vi "read station LIN config.vi"(0 "configuration file path in":path, 1 "lin channel count":i32=1, 5 "station idx":i32, 9 "ldf file name":string="CD701_CEM_LIN3_20230222", 11 "error in":errorcluster, 12 "NAD":u8) -> (3 "XNET LIN":bool, 4 "configuration file path out":path, 8 "LIN INFO":T1={"Toolkit Type"=enum."Inalfa LIN", "NAD"=36, "Inalfa LIN"={"Master Frame(3C)"="MasterReq\nSPA3414_ConfigurationsCMAGeely_CEMCALYPSOSDB34XX0Cfg_LIN3_190709_", "Slave Frame(3D)"="SlaveResp\nSPA3414_ConfigurationsCMAGeely_CEMCALYPSOSDB34XX0Cfg_LIN3_190709_", "Request Schedule"="CEMLIN3DiagRequestSchedule\nSPA3414_ConfigurationsCMAGeely_CEMCALYPSOSDB34XX0Cfg_LIN3_190709_", "Response Schedule"="CEMLIN3DiagResponseSchedule\nSPA3414_ConfigurationsCMAGeely_CEMCALYPSOSDB34XX0Cfg_LIN3_190709_", "Frame Write SCU"="", "Frame Read SCU"="", "LIN Name"=""}, "ADCS LIN"={"Port"="", "HW select"=0, "XNET Cluster"="NIXNET_exampleLDF", "ByteCmd Path"=path "C:/Labview Code/System/ByteCmdConfig.txt"}, "TS LIN"={"ref info"=refnum, "LIN Channel"=0, "ByteCmd Path"=path "C:/Labview Code/System/ByteCmdConfig.txt"}} {"NAD" format="%.0x"; "ADCS LIN"."HW select" items=["NI-XNET", "NI-CAN"]}, 15 "error out":errorcluster)   [LabVIEW 2018]
uses:
  02.Type Def's/station LIN config.ctl
  03.Inalfa LIN/LIN Device.ctl
  <vilib>/CMC.AME/Inalfa ADCS/Ctl'Def/ADCS_LIN info.ctl
  C:/Program Files (x86)/National Instruments/LabVIEW 2018/vi.lib/CMC.AME/Inalfa TS LIN/TOSUN/TSMaster/bin/Interop.TSMasterAPI.dll
  Program Files (x86)/National Instruments/LabVIEW 2018/vi.lib/CMC.AME/Inalfa TS LIN/TOSUN/TSMaster/bin/Interop.TSMasterAPI.dll
  05.UserVI's/file io/ini/type defs/ini file actions.ctl
  05.UserVI's/file io/ini/type defs/ini entry types.ctl
  05.UserVI's/file io/ini/type defs/ini entry.ctl
  05.UserVI's/file io/ini/type defs/ini entry value.ctl
panel:
  out "LIN Device Name":string
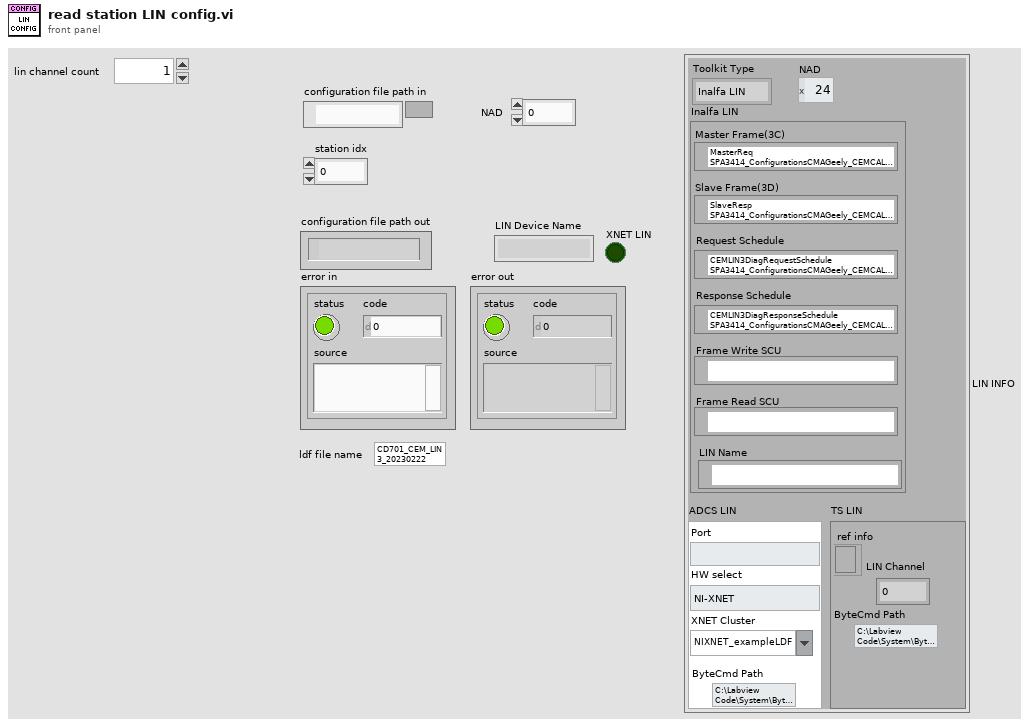
[diagram p1: front panel]
types:
  T1 = typedef "station LIN config.ctl" = cluster{"Toolkit Type":enum16{"Inalfa LIN", "ADCS LIN", "TS LIN"}, "NAD":u8, "Inalfa LIN":T2, "ADCS LIN":T3, "TS LIN":cluster{"ref info":refnum<k24>, "LIN Channel":i32, "ByteCmd Path":path}}
  T2 = typedef "LIN Device.ctl" = cluster{"Master Frame(3C)":refnum<k21>, "Slave Frame(3D)":refnum<k21>, "Request Schedule":refnum<k21>, "Response Schedule":refnum<k21>, "Frame Write SCU":refnum<k21>, "Frame Read SCU":refnum<k21>, "LIN Name":refnum<k21>}
  T3 = typedef "ADCS_LIN info.ctl" = cluster{"Port":string, "HW select":u16, "XNET Cluster":string, "ByteCmd Path":path}
  T4 = typedef "ini file actions.ctl" = enum16{"read ini", "write ini"}
  T5 = typedef "ini entry.ctl" = cluster{"section":string, "key":string, "type":T6, "default value":T7}
  T6 = typedef "ini entry types.ctl" = enum16{"Boolean", "Double", "I32", "Path", "String", "U32"}
  T7 = typedef "ini entry value.ctl" = cluster{"Boolean":bool, "Dbl":dbl, "I32":i32, "Path":path, "String":string, "U32":u32}
  T8 = cluster{"status":bool, "code":i32, "error desp":string}
  T9 = cluster{"Ref out":refnum<k24>, "station idx":i32, "appended path":path}
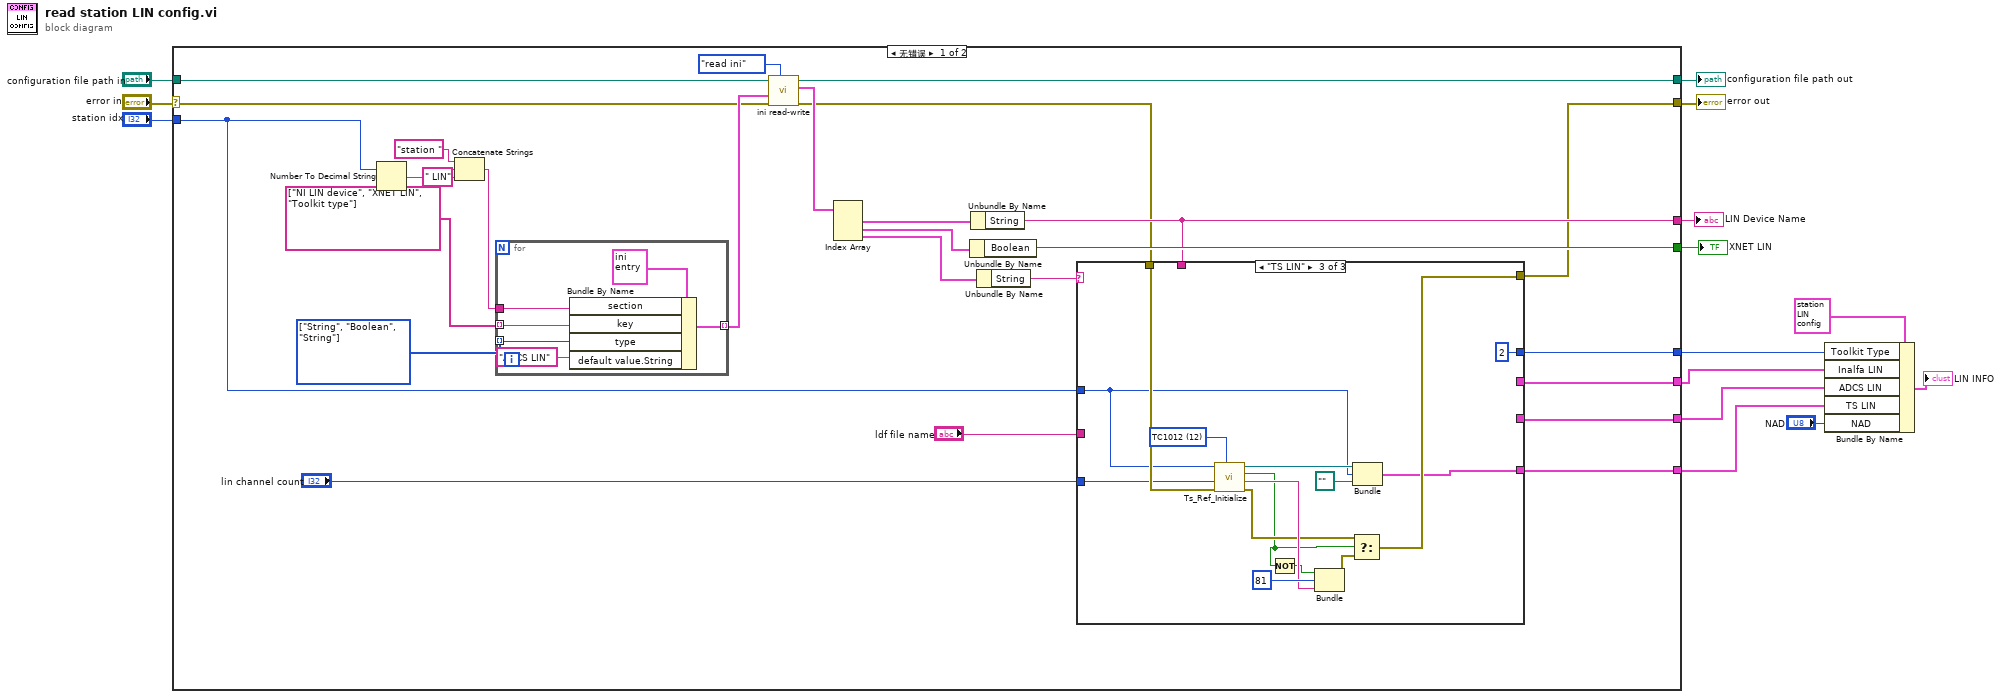
[diagram p0: block diagram]
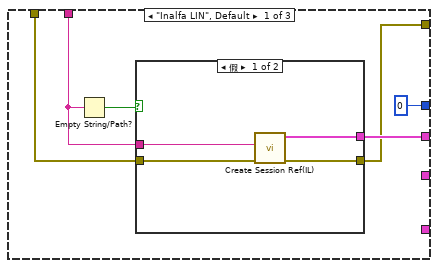
[diagram p2: hidden frame]
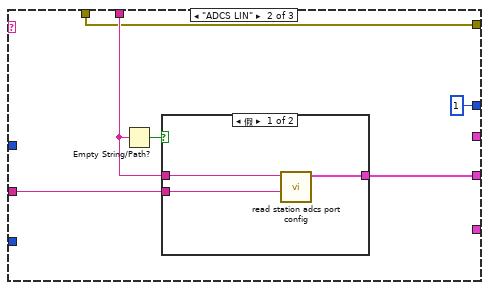
[diagram p4: hidden frame]
diagram:
  n1 = case shown="无错误" "error in" {
    selector: "error in" -> [w32 w84]
    tunnel: "configuration file path in" -> [w41 w83]
    tunnel: [w18 w83] -> w13
    tunnel: [w22 w84] -> w12
    tunnel: "station idx" -> [w16 _]
    tunnel: [w25 _] -> w9
    tunnel: [w28 _] -> w8
    tunnel: [w24 _] -> w6
    tunnel: [w21 _] -> w5
    tunnel: [w19 _] -> w2
    tunnel: [w17 _] -> w3
    frame No Error {
      w34 = T6[] [enum."String", enum."Boolean", enum."String"] items=["Boolean", "Double", "I32", "Path", "String", "U32"]
      n2 = Number To Decimal String(number=w16) -> (decimal integer string=w37:string)  [unwired: 1 in]
      n3 = Concatenate Strings("station ", w37, " LIN" ("string")) -> (w36:string)
      n4 = for {
        tunnel: w36 -> [w81]
        tunnel: string[] ["NI LIN device", "XNET LIN", "Toolkit type"] -> [w80] mode=indexing
        tunnel: w34 -> [w79] mode=indexing
        tunnel: [w78] -> w33 mode=indexing
        n5 = Bundle By Name(cluster=T5 {"section"="", "key"="", "type"=enum."Boolean", "default value"={"Boolean"=FALSE, "Dbl"=0.0, "I32"=0, "Path"=path "", "String"="", "U32"=0}}, "section"=w81, "key"=w80, "type"=w79, "default value.String"="ADCS LIN") -> (w78:T5)
      }
      n6 = call "ini read-write.vi"("action"=ini_file_actions."read ini", "error in (no error)"=w32, "ini entry descriptors"=w33, "configuration file path"=w41) -> ("error out"=w23:errorcluster, "values out"=w39:T7[], "configuration file path out"=w18:path)  [unwired: 5 in]
      n7 = Index Array(array=w39) -> (element #1=w30:T7, element #2=w29:T7, element #3=w27:T7)  [unwired: 3 in]
      n8 = Unbundle By Name(w29) -> ("Boolean"=w28:bool)
      n9 = Unbundle By Name(w30) -> ("String"=w25:string)
      n10 = Unbundle By Name(w27) -> ("String"=w26:string)
      n11 = case shown="\"TS LIN\"" w26 {
        tunnel: w25 -> [w46 w58 _]
        tunnel: [w47 _ _] -> w24
        tunnel: w23 -> [w44 w54 w68]
        tunnel: [w43 w54 w73] -> w22
        tunnel: [_ w56 _] -> w21
        tunnel: "ldf file name" -> [_ w55 _]
        tunnel: [_ _ w71] -> w19
        tunnel: [0 1 2] -> w17
        tunnel: w16 -> [_ _ w62]
        tunnel: "lin channel count" -> [_ _ w63]
        frame "Inalfa LIN", Default {
          n12 = Empty String/Path?(string/path=w46) -> (empty?=w45:bool)
          n13 = case shown="假" w45 {
            tunnel: w46 -> [w51 _]
            tunnel: [w50 _] -> w47
            tunnel: w44 -> [w49 w52]
            tunnel: [w48 w52] -> w43
            frame False {
              n14 = call "Create Session Ref(IL).vi"("error in (no error)"=w49, "interface"=w51) -> ("error out"=w48:errorcluster, "LIN Device"=w50:T2)  [unwired: 8 in]
            }
            frame True {
            }
          }
        }
        frame "ADCS LIN" {
          n15 = Empty String/Path?(string/path=w58) -> (empty?=w57:bool)
          n16 = case shown="假" w57 {
            tunnel: w58 -> [w61 _]
            tunnel: [w60 _] -> w56
            tunnel: w55 -> [w59 _]
            frame False {
              n17 = call "read station adcs port config.vi"("ldf file name"=w59, "port"=w61) -> ("ADCS LIN"=w60:T3)  [unwired: 9 in]
            }
            frame True {
            }
          }
        }
        frame "TS LIN" {
          w64 = 12 items=["TS_UNKNOWN_DEVICE"=0, "TC1001 "=3, "TL1001"=4, "TC1011"=5, "TC1002"=7, "TC1014"=8, "TC1026"=10, "TC1016"=11, "TC1012"=12, "TC1013 "=13, "TC1034"=15, "TP1026"=31] ("FHWDeviceSubType")
          n18 = call <vilib>:"Ts_Ref_Initialize.vi"("FHWDeviceSubType"=w64, "error in"=w68, "lin channel count"=w63, "AIdxChn"=w62) -> ("error out"=w67:errorcluster, "error desp"=w75:string, "pass?"=w65:bool, "Ref out"=w72:refnum<k24>)  [unwired: 4 in]
          n19 = Not(x=w65) -> (.not. x?=w66:bool)
          n20 = Bundle(w66, 81, "error desp"=w75) -> (w74:cluster{bool, i32, "error desp":string})  [unwired: 1 in]
          n21 = Select(t=w67, s=w65, f=w74) -> (s? t:f=w73:T8)
          n22 = Bundle("Ref out"=w72, "station idx"=w62, "appended path"=path "") -> (w71:T9)  [unwired: 1 in]
        }
      }
    }
    frame Error {
    }
  }
  "configuration file path out" <- w13
  "error out" <- w12
  "LIN Device Name" <- w9
  "XNET LIN" <- w8
  n23 = Bundle By Name(cluster=T1 {"Toolkit Type"=enum."Inalfa LIN", "NAD"=36, "Inalfa LIN"={"Master Frame(3C)"="MasterReq\nSPA3414_ConfigurationsCMAGeely_CEMCALYPSOSDB34XX0Cfg_LIN3_190709_", "Slave Frame(3D)"="SlaveResp\nSPA3414_ConfigurationsCMAGeely_CEMCALYPSOSDB34XX0Cfg_LIN3_190709_", "Request Schedule"="CEMLIN3DiagRequestSchedule\nSPA3414_ConfigurationsCMAGeely_CEMCALYPSOSDB34XX0Cfg_LIN3_190709_", "Response Schedule"="CEMLIN3DiagResponseSchedule\nSPA3414_ConfigurationsCMAGeely_CEMCALYPSOSDB34XX0Cfg_LIN3_190709_", "Frame Write SCU"="", "Frame Read SCU"="", "LIN Name"=""}, "ADCS LIN"={"Port"="", "HW select"=0, "XNET Cluster"="NIXNET_exampleLDF", "ByteCmd Path"=path "C:/Labview Code/System/ByteCmdConfig.txt"}, "TS LIN"={"ref info"=refnum, "LIN Channel"=0, "ByteCmd Path"=path "C:/Labview Code/System/ByteCmdConfig.txt"}} ("LIN INFO"), "Toolkit Type"=w3, "Inalfa LIN"=w6, "ADCS LIN"=w5, "TS LIN"=w2, "NAD"="NAD") -> (→"LIN INFO":T1)
